vi "Receiver.vi"() -> (0 "Channel 7 position":u8, 1 "Channel 6 position":u8, 2 "Channel 5 position":u8, 3 "Channel 4 position":u8, 4 "Value Channel 0":i32, 5 "Value Channel 2":i32, 7 "Value Channel 3":i32)   [LabVIEW 2016]
doc: "Inputs\n-\n\nOutputs\nPosition for channel 4, 5, 6, 7\nValue channel 0\n\nThis VI reads the signals from the RC receiver, process the data and outputs the position on the switches (channel 4. 5, 6, 7) and the value for channel 0 which corresponds to the horisontal positon of the right joystick."
uses:
  <vilib>/rvi/Emulation/niFpgaGetClockAttributes.vi
  <vilib>/rvi/Emulation/niFpgaSctlEmulationGetInTimedLoop.vi
  <vilib>/rvi/Emulation/niFpgaEmulationReportErrorSimple.vi
  <vilib>/rvi/eio/common/nirviEmuTemplateMethod_errors.vi
  <vilib>/rvi/Emulation/niFpgaCriticalErrorInLSC.vi
  <vilib>/eio/EIONode/EIONode.xnode
panel:
  in  "Sync Pulse Max":u32=15000
  in  "Sync Pulse Min":u32=3500
  out "Value Channel 1":u32
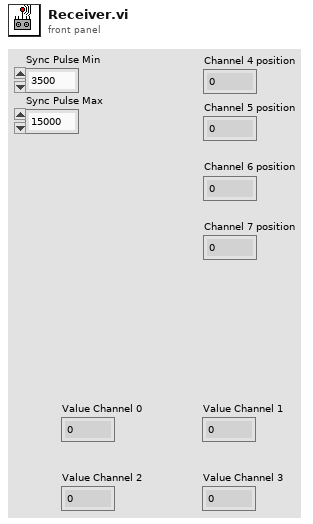
[diagram p1: front panel]
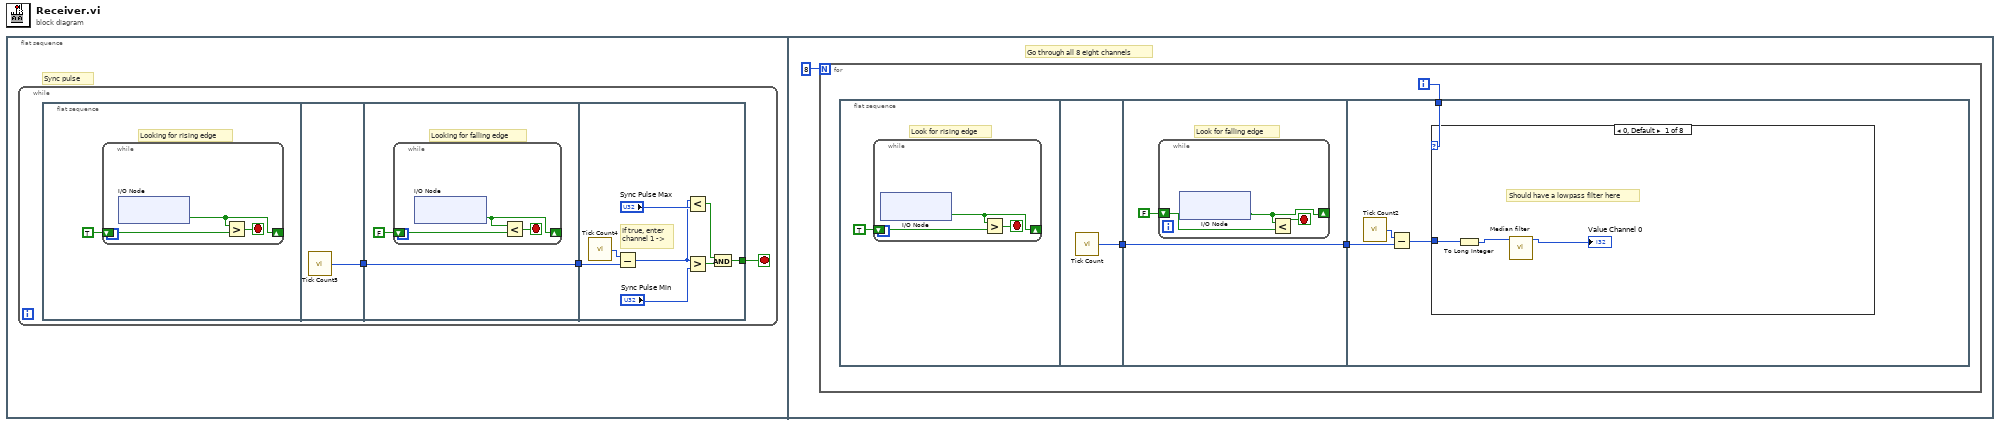
[diagram p0: block diagram]
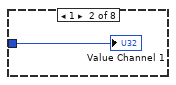
[diagram p2: hidden frame]
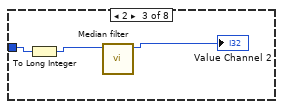
[diagram p3: hidden frame]
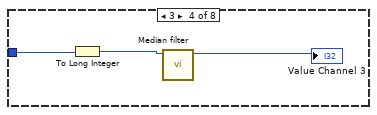
[diagram p4: hidden frame]
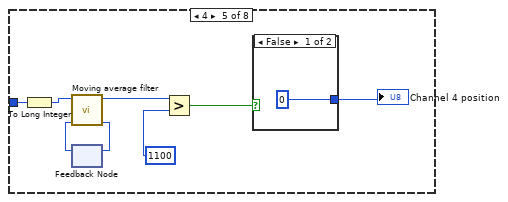
[diagram p5: hidden frame]
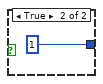
[diagram p6: hidden frame]
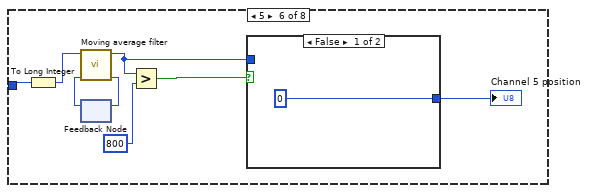
[diagram p7: hidden frame]
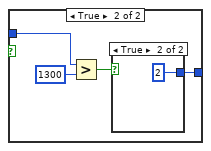
[diagram p8: hidden frame]
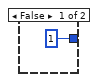
[diagram p9: hidden frame]
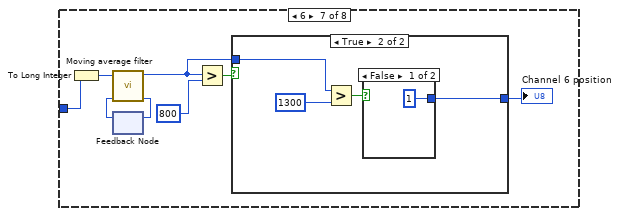
[diagram p10: hidden frame]
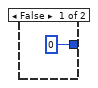
[diagram p11: hidden frame]
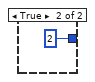
[diagram p12: hidden frame]
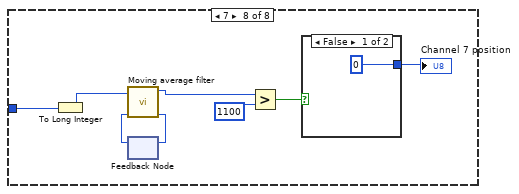
[diagram p13: hidden frame]
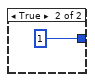
[diagram p14: hidden frame]
diagram:
  n1 = flat-sequence {
    frame #0 {
      # "Sync pulse"
      n2 = while {
        stop <- w1 stop-if-true
        n3 = flat-sequence {
          tunnel: [w8] -> w3
          tunnel: w3 -> [w9]
          tunnel: [w9] -> w2
          tunnel: [w21] -> w1
          tunnel: w2 -> [w16]
          frame #0 {
            # "Looking for rising edge"
            n4 = while {
              shift-right: [w5] -> _
              shift-left: TRUE -> [w6]
              stop <- w7 stop-if-true
              n5 = xnode "I/O Node"() -> ("DIO/DIO4"=w5:bool)  [unwired: 1 in, 1 out]
              n6 = Greater?(x=w5, y=w6) -> (0:w7:bool)
            }
          }
          frame #1 {
            n7 = call "Tick Count5"() -> ("Tick Count(uSec)"=w8:u32)
          }
          frame #2 {
            # "Looking for falling edge"
            n8 = while {
              shift-right: [w11] -> _
              shift-left: FALSE -> [w12]
              stop <- w13 stop-if-true
              n9 = xnode "I/O Node"() -> ("DIO/DIO4"=w11:bool)  [unwired: 1 in, 1 out]
              n10 = Less?(x=w11, y=w12) -> (x < y?=w13:bool)
            }
          }
          frame #3 {
            # "If true, enter \nchannel 1 ->"
            n11 = call "Tick Count4"() -> ("Tick Count(uSec)"=w17:u32)
            n12 = Subtract(x=w17, y=w16) -> (x-y=w14:u32)
            n13 = Less?(x=w14, y="Sync Pulse Max") -> (x < y?=w19:bool)
            n14 = Greater?(x=w14, y="Sync Pulse Min") -> (0:w20:bool)
            n15 = And(x=w19, y=w20) -> (x .and. y?=w21:bool)
          }
        }
      }
    }
    frame #1 {
      # "Go through all 8 eight channels"
      n16 = for {
        N: 8 -> [_]
        i -> [w23]
        n17 = flat-sequence {
          tunnel: [w30] -> w25
          tunnel: [w31] -> w24
          tunnel: w25 -> [w31]
          tunnel: w23 -> [w39]
          tunnel: w24 -> [w37]
          frame #0 {
            # "Look for rising edge"
            n18 = while {
              shift-right: [w27] -> _
              shift-left: TRUE -> [w28]
              stop <- w29 stop-if-true
              n19 = xnode "I/O Node"() -> ("DIO/DIO4"=w27:bool)  [unwired: 1 in, 1 out]
              n20 = Greater?(x=w27, y=w28) -> (0:w29:bool)
            }
          }
          frame #1 {
            n21 = call "Tick Count"() -> ("Tick Count(uSec)"=w30:u32)
          }
          frame #2 {
            # "Look for falling edge"
            n22 = while {
              shift-right: [w33] -> _
              shift-left: FALSE -> [w34]
              stop <- w35 stop-if-true
              n23 = xnode "I/O Node"() -> ("DIO/DIO4"=w33:bool)  [unwired: 1 in, 1 out]
              n24 = Less?(x=w33, y=w34) -> (x < y?=w35:bool)
            }
          }
          frame #3 {
            n25 = call "Tick Count2"() -> ("Tick Count(uSec)"=w38:u32)
            n26 = Subtract(x=w38, y=w37) -> (x-y=w36:u32)
            n27 = case shown="0, Default" w39 {
              tunnel: w36 -> [w41 w43 w46 w49 w51 w60 w76 w91]
              frame 0, Default {
                # "Should have a lowpass filter here"
                n28 = To Long Integer(number=w41) -> (32bit integer=w40:i32)
                n29 = call "Median filter.vi"("Rawdata"=w40) -> ("Filtered element"=→"Value Channel 0":i32)  [unwired: 10 in]
              }
              frame 1 {
                "Value Channel 1" <- w43
              }
              frame 2 {
                n30 = To Long Integer(number=w46) -> (32bit integer=w45:i32)
                n31 = call "Median filter.vi"("Rawdata"=w45) -> ("Filtered element"=→"Value Channel 2":i32)  [unwired: 10 in]
              }
              frame 3 {
                n32 = To Long Integer(number=w49) -> (32bit integer=w48:i32)
                n33 = call "Median filter.vi"("Rawdata"=w48) -> ("Filtered element"=→"Value Channel 3":i32)  [unwired: 10 in]
              }
              frame 4 {
                n34 = To Long Integer(number=w51) -> (32bit integer=w50:i32)
                n35 = feedback #1() -> (w53:i32)  [unwired: 1 in]
                n36 = call "Moving average filter.vi"("x"=w53, "Input"=w50) -> ("xdot"=w52:i32, "Mean"=w54:i32)  [unwired: 8 in]
                n37 = feedback-in #1(w52) -> ()
                n38 = Greater?(x=w54, y=1100) -> (0:w56:bool)
                n39 = case shown="False" w56 {
                  tunnel: [u8 0 u8 1] -> w55
                  frame False {
                  }
                  frame True {
                  }
                }
                "Channel 4 position" <- w55
              }
              frame 5 {
                n40 = To Long Integer(number=w60) -> (32bit integer=w61:i32)
                n41 = feedback #2() -> (w65:i32)  [unwired: 1 in]
                n42 = call "Moving average filter.vi"("x"=w65, "Input"=w61) -> ("xdot"=w64:i32, "Mean"=w63:i32)  [unwired: 8 in]
                n43 = feedback-in #2(w64) -> ()
                n44 = Greater?(x=w63, y=800) -> (0:w67:bool)
                n45 = case shown="False" w67 {
                  tunnel: w63 -> [_ w71]
                  tunnel: [u8 0 w69] -> w66
                  frame False {
                  }
                  frame True {
                    n46 = Greater?(x=w71, y=1300) -> (0:w72:bool)
                    n47 = case shown="True" w72 {
                      tunnel: [u8 1 u8 2] -> w69
                      frame False {
                      }
                      frame True {
                      }
                    }
                  }
                }
                "Channel 5 position" <- w66
              }
              frame 6 {
                n48 = To Long Integer(number=w76) -> (32bit integer=w75:i32)
                n49 = feedback #3() -> (w79:i32)  [unwired: 1 in]
                n50 = call "Moving average filter.vi"("x"=w79, "Input"=w75) -> ("xdot"=w78:i32, "Mean"=w77:i32)  [unwired: 8 in]
                n51 = feedback-in #3(w78) -> ()
                n52 = Greater?(x=w77, y=800) -> (0:w81:bool)
                n53 = case shown="True" w81 {
                  tunnel: w77 -> [_ w86]
                  tunnel: [u8 0 w85] -> w82
                  frame False {
                  }
                  frame True {
                    n54 = Greater?(x=w86, y=1300) -> (0:w87:bool)
                    n55 = case shown="False" w87 {
                      tunnel: [u8 1 u8 2] -> w85
                      frame False {
                      }
                      frame True {
                      }
                    }
                  }
                }
                "Channel 6 position" <- w82
              }
              frame 7 {
                n56 = To Long Integer(number=w91) -> (32bit integer=w90:i32)
                n57 = feedback #4() -> (w93:i32)  [unwired: 1 in]
                n58 = call "Moving average filter.vi"("x"=w93, "Input"=w90) -> ("xdot"=w92:i32, "Mean"=w94:i32)  [unwired: 8 in]
                n59 = feedback-in #4(w92) -> ()
                n60 = Greater?(x=w94, y=1100) -> (0:w97:bool)
                n61 = case shown="False" w97 {
                  tunnel: [u8 0 u8 1] -> w95
                  frame False {
                  }
                  frame True {
                  }
                }
                "Channel 7 position" <- w95
              }
            }
          }
        }
      }
    }
  }
